vi "Boolean Operation.vi"(1 "B":bool, 2 "A":bool) -> (0 "AandB":bool)   [LabVIEW 2012]
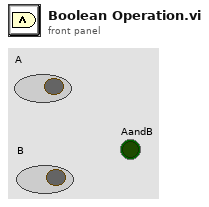
[diagram p1: front panel]
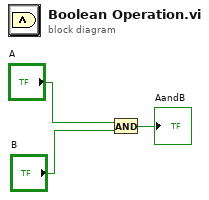
[diagram p0: block diagram]
diagram:
  n1 = And(x="A", y="B") -> (x .and. y?=→"AandB":bool)
